vi "String to DTItem.vi"(7 "image path":path, 8 "error in (no error)":errorcluster, 10 "datatype":T1, 11 "element":string) -> (0 "error out":errorcluster, 3 "DTItem .NET Refnum out":refnum<k24>)   [LabVIEW 2016, in "DataGrid.lvlib" / "DataTable.lvclass"]
uses:
  <userlib>/LabVIEWdotNetDataGrid/source/DataTable/DataTable.lvclass
  <userlib>/LabVIEWdotNetDataGrid/source/GridColumn/ColumnType.ctl
  <userlib>/LabVIEWdotNetDataGrid/source/GridColumn/GridColumn.lvclass
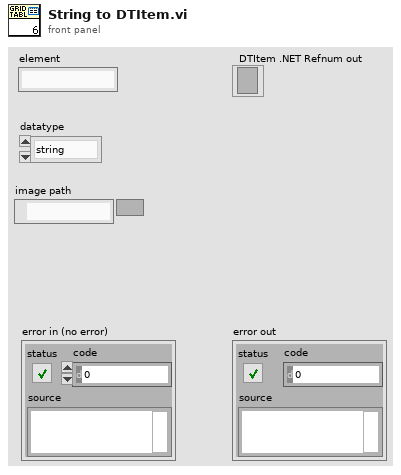
[diagram p1: front panel]
types:
  T1 = typedef "DataGrid.lvlib/GridColumn.lvclass/ColumnType.ctl" = enum16{"string", "image", "check", "numeric", "timestamp", "button", "combo", "link"}
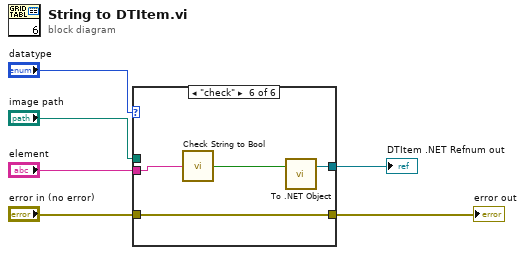
[diagram p0: block diagram]
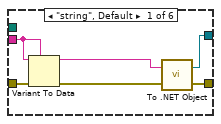
[diagram p2: hidden frame]
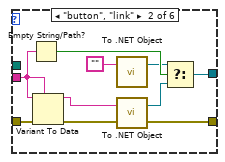
[diagram p3: hidden frame]
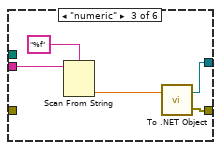
[diagram p4: hidden frame]
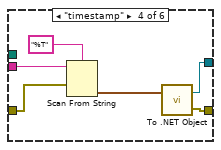
[diagram p5: hidden frame]
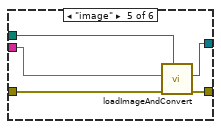
[diagram p6: hidden frame]
diagram:
  n1 = case shown="\"check\"" "datatype" {
    tunnel: "element" -> [w8 w18 w25 w31 w38 w40]
    tunnel: [w7 w15 w26 w32 w37 w41] -> w2
    tunnel: "error in (no error)" -> [w11 w21 _ w29 w36 w42]
    tunnel: [w9 w19 w27 w33 w35 w42] -> w4
    tunnel: "image path" -> [_ _ _ _ w34 _]
    frame "string", Default {
      n2 = Variant To Data(error in=w11, type=w8, Variant=w8) -> (data=w12:string, error out=w10:errorcluster)
      n3 = call <vilib>:"To .NET Object.vi"("error in (no error)"=w10, "anything"=w12) -> ("error out"=w9:errorcluster, ".NET object"=w7:refnum<k24>)
    }
    frame "button", "link" {
      n4 = Empty String/Path?(string/path=w18) -> (empty?=w17:bool)
      n5 = Variant To Data(error in=w21, type=w18, Variant=w18) -> (data=w22:string, error out=w20:errorcluster)
      n6 = call <vilib>:"To .NET Object.vi"("anything"="") -> (".NET object"=w13:refnum<k24>)  [unwired: 1 in, 1 out]
      n7 = call <vilib>:"To .NET Object.vi"("error in (no error)"=w20, "anything"=w22) -> ("error out"=w19:errorcluster, ".NET object"=w16:refnum<k24>)
      n8 = Select(t=w13, s=w17, f=w16) -> (s? t:f=w15:refnum<k24>)
    }
    frame "numeric" {
      n9 = Scan From String(format string="%f", input string=w25) -> (output 1=w23:dbl)  [unwired: 3 in, 3 out]
      n10 = call <vilib>:"To .NET Object.vi"("anything"=w23) -> ("error out"=w27:errorcluster, ".NET object"=w26:refnum<k24>)  [unwired: 1 in]
    }
    frame "timestamp" {
      n11 = Scan From String(format string="%T", input string=w31, error in=w29) -> (output 1=w28:timestamp)  [unwired: 2 in, 3 out]
      n12 = call <vilib>:"To .NET Object.vi"("anything"=w28) -> ("error out"=w33:errorcluster, ".NET object"=w32:refnum<k24>)  [unwired: 1 in]
    }
    frame "image" {
      n13 = call <userlib>:"loadImageAndConvert.vi"("image path"=w34, "error in (no error)"=w36, "name or relative path"=w38) -> ("error out"=w35:errorcluster, ".NET object"=w37:refnum<k24>)  [unwired: 7 in]
    }
    frame "check" {
      n14 = call <userlib>:"Check String to Bool.vi"("string of check"=w40) -> ("Boolean"=w39:bool)
      n15 = call <vilib>:"To .NET Object.vi"("anything"=w39) -> (".NET object"=w41:refnum<k24>)  [unwired: 1 in, 1 out]
    }
  }
  "error out" <- w4
  "DTItem .NET Refnum out" <- w2
